vi "14 Function Generator Signal (x64-2018).vi"(8 "Error In":errorcluster, 9 "Rate":dbl=1000.0, 10 "Number of samples per channel":dbl=40.0, 11 "task/channels in":refnum<k21>) -> (0 "Error Out":errorcluster, 2 "data":waveform(dbl)[](array[waveform]), 3 "task out":refnum<k21>)   [LabVIEW 2017]
uses:
  <vilib>/DAQmx/read.llb/DAQmx Read (Analog 1D Wfm NChan NSamp Duration).vi
  <vilib>/DAQmx/create/channels.llb/DAQmx Create Channel (AI-Voltage-Basic).vi
  <vilib>/DAQmx/configure/timing.llb/DAQmx Timing (Sample Clock).vi
  <vilib>/DAQmx/miscellaneous.llb/DAQmx Fill In Error Info.vi
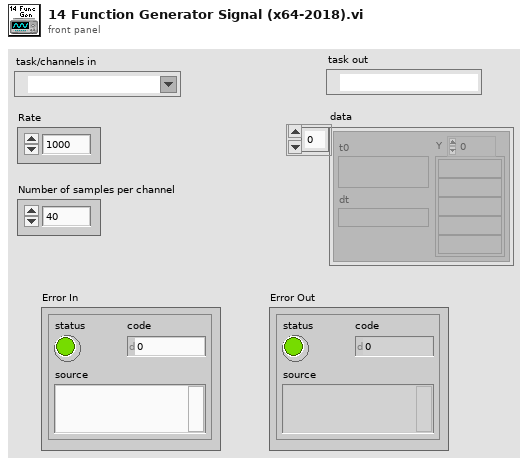
[diagram p1: front panel]
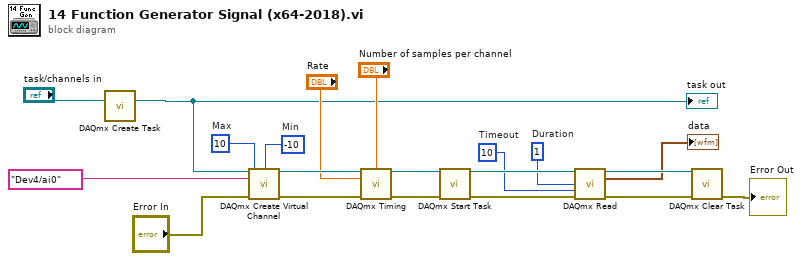
[diagram p0: block diagram]
diagram:
  w15 = 1  # Duration
  w16 = 10  # Timeout
  w20 = 10  # Max
  w19 = -10  # Min
  n1 = call <vilib>:"DAQmx Create Task.vi"("task to copy"="task/channels in") -> ("task out"=w3:refnum<k21>)  [unwired: 13 in, 1 out]
  "task out" <- w3
  n2 = call-poly <vilib>:"DAQmx Create Virtual Channel.vi"("task in"=w3, "maximum value"=w20, "minimum value"=w19, "physical channels"=tag "Dev4/ai0" ("DAQmx Physical Channel"), "error in"="Error In") -> ("task out"=w14:refnum<k21>, "error out"=w12:errorcluster)  [unwired: 9 in]
  n3 = call-poly <vilib>:"DAQmx Timing.vi"("task/channels in"=w14, "samples per channel"="Number of samples per channel", "rate"="Rate", "error in"=w12) -> ("task out"=w13:refnum<k21>, "error out"=w11:errorcluster)  [unwired: 10 in]
  n4 = call <vilib>:"DAQmx Start Task.vi"("task/channels in"=w13, "error in"=w11) -> ("task out"=w18:refnum<k21>, "error out"=w17:errorcluster)  [unwired: 12 in]
  n5 = call-poly <vilib>:"DAQmx Read.vi"("task/channels in"=w18, "duration"=w15, "timeout"=w16, "error in"=w17) -> ("task out"=w10:refnum<k21>, "data"=→"data":waveform(dbl)[], "error out"=w9:errorcluster)  [unwired: 9 in]
  n6 = call <vilib>:"DAQmx Clear Task.vi"("task in"=w10, "error in"=w9) -> ("error out"=→"Error Out":errorcluster)  [unwired: 13 in]
